vi "Preview the image.vi"() -> ()   [LabVIEW 2018]
uses:
  <userlib>/LabViewDVPCamera/LabViewDVPCamera.lvlib
panel:
  in  "CloseFlg":i32
  out "handle":u32
  out "new picture":picture caption="新图片"
  in  "CameraList":u16(ring) items=["USB2_3M(19)@1112121"]
  in  "Set":bool
  in  "Close":bool
  in  "Open":bool
  in  "ScanCamera":bool
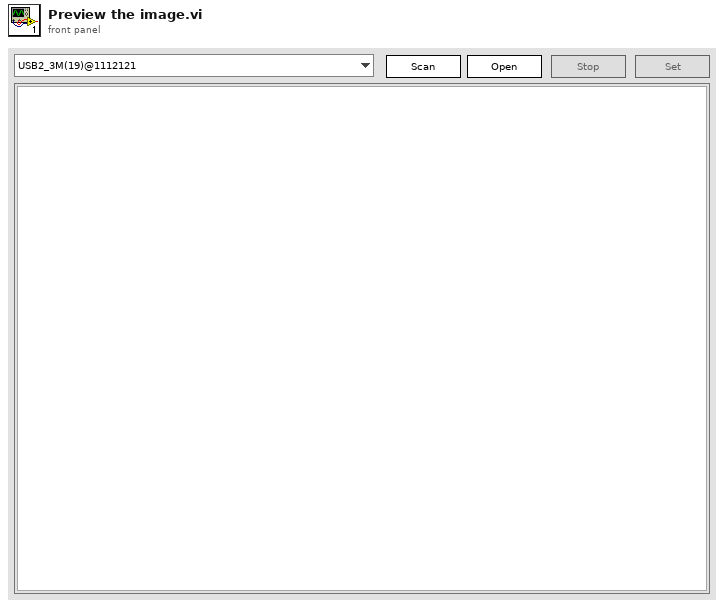
[diagram p1: front panel]
types:
  T1 = enum8{"Enabled", "Disabled", "Disabled and Grayed Out"}
  T2 = typedef "LVStringsAndValuesArrayTypeDef_U16.ctl" = cluster{"String":string, "Value":u16}[]
  T3 = cluster{"image type":i16, "image depth":u8, u8[], "无符号8位数组":u8[], u32[], cluster{u16, u16, u16, u16}}
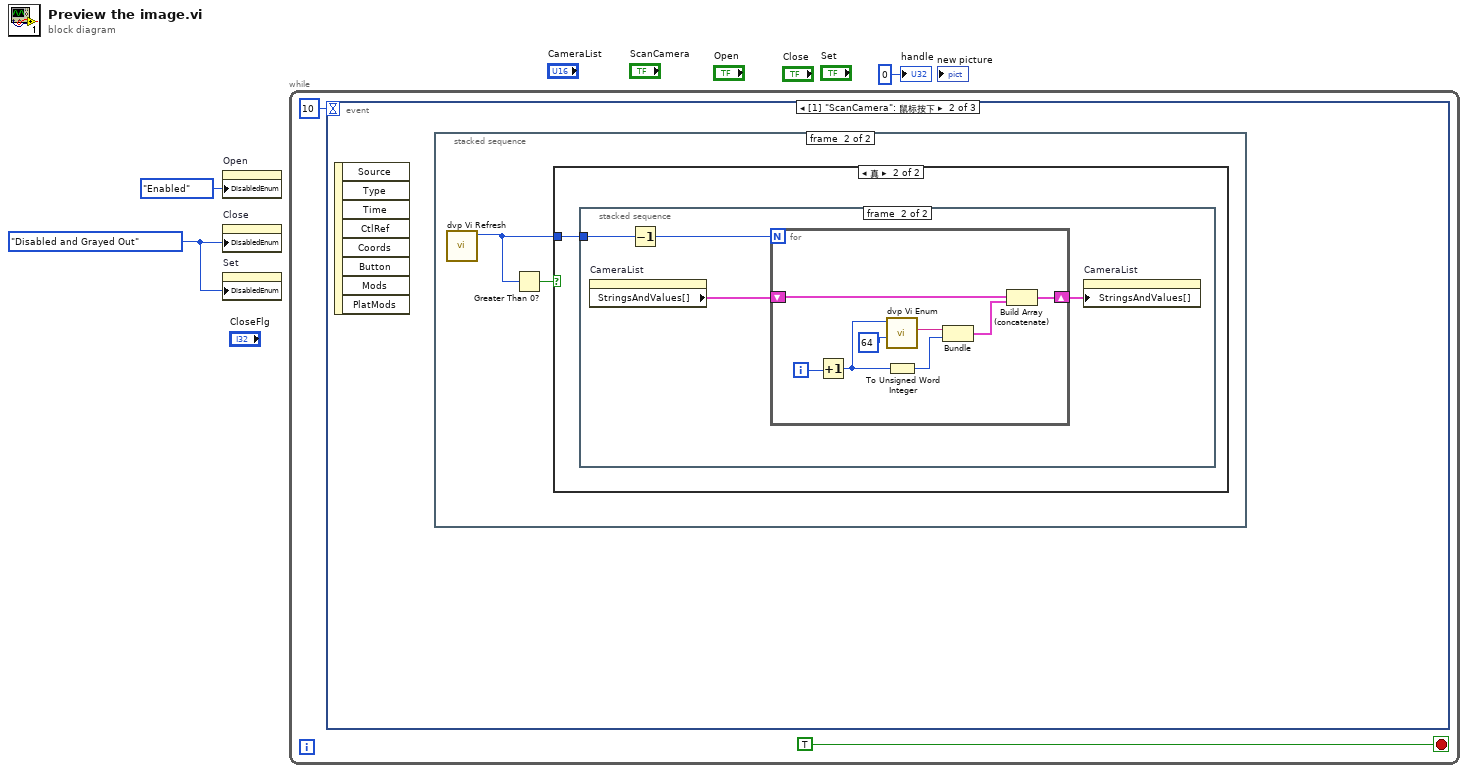
[diagram p0: block diagram]
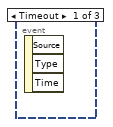
[diagram p2: hidden frame]
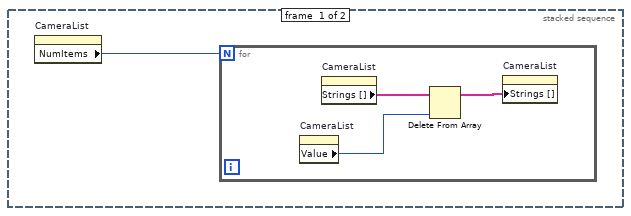
[diagram p3: hidden frame]
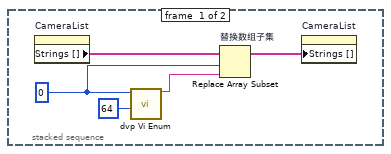
[diagram p5: hidden frame]
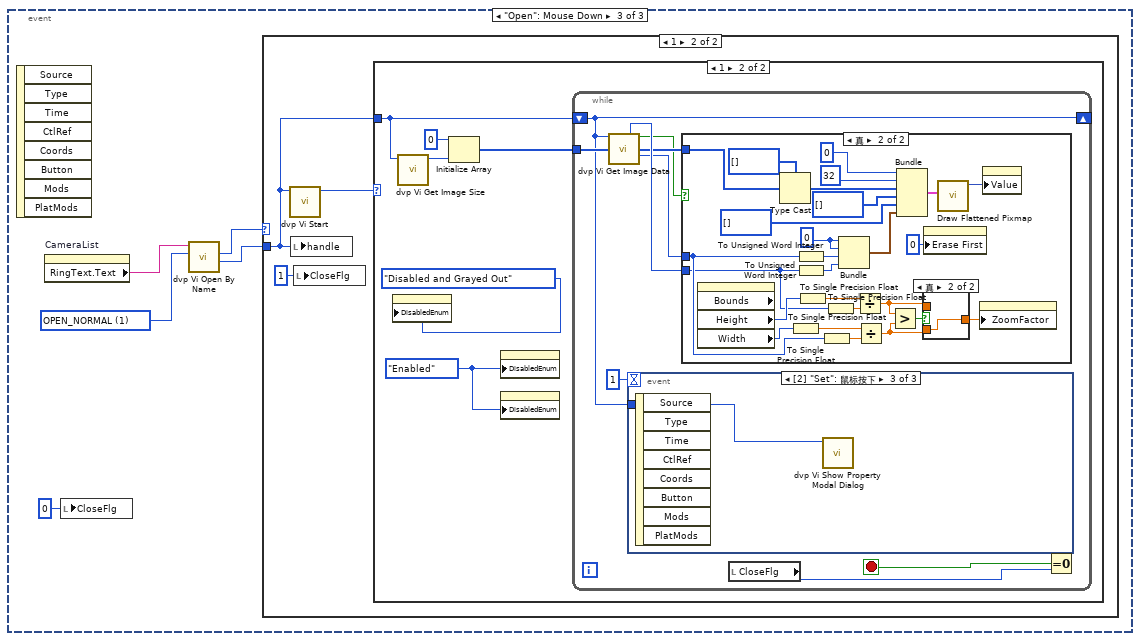
[diagram p6: hidden frame]
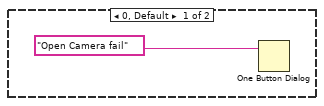
[diagram p7: hidden frame]
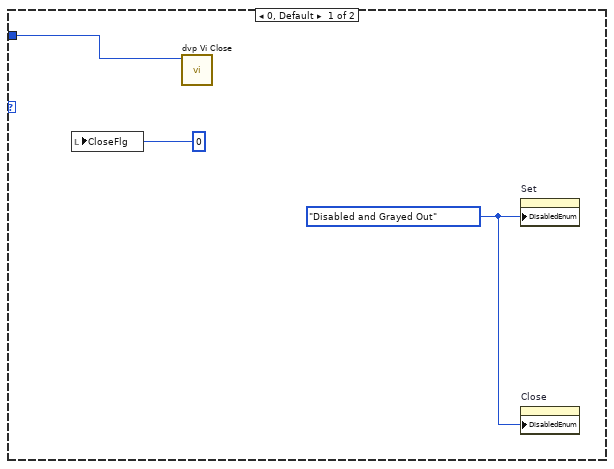
[diagram p8: hidden frame]
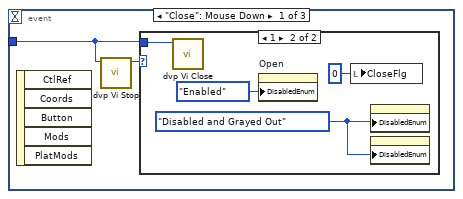
[diagram p9: hidden frame]
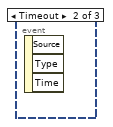
[diagram p11: hidden frame]
diagram:
  w2 = T1."Disabled and Grayed Out" ("禁用")
  n1 = property on="Open" class="Bool"("DisabledEnum"=T1."Enabled" ("禁用")) -> ()  [unwired: 2 in, 2 out]
  n2 = property on="Close" class="Bool"("DisabledEnum"=w2) -> ()  [unwired: 2 in, 2 out]
  n3 = property on="Set" class="Bool"("DisabledEnum"=w2) -> ()  [unwired: 2 in, 2 out]
  n4 = while {
    stop <- TRUE stop-if-true
    n5 = event shown="[1] \"ScanCamera\": 鼠标按下" {
      selector: _ -> [_ _ _]
      dyn-events: _ -> [_ _ _]
      timeout: 10 -> [_ _ _]
      event Timeout {
        n6 = event-data() -> ()  [unwired: 1 in, 3 out]
      }
      event "ScanCamera": Mouse Down {
        n7 = event-data() -> ()  [unwired: 1 in, 8 out]
        n8 = stacked-sequence "清除下拉列表的数据" {
          frame #0 {
            n9 = property on="CameraList" class="Ring (严格)"() -> ("NumItems"=w6:u32)  [unwired: 2 in, 2 out]
            n10 = for {
              N: w6 -> [_]
              n11 = property on="CameraList" class="Ring (严格)"() -> ("Value"=w8:u16)  [unwired: 2 in, 2 out]
              n12 = property on="CameraList" class="Ring (严格)"() -> ("Strings []"=w7:string[])  [unwired: 2 in, 2 out]
              n13 = Delete From Array ("删除数组元素")(array=w7, index=w8) -> (array with subset deleted=w9:string[])  [unwired: 1 in, 1 out]
              n14 = property on="CameraList" class="Ring (严格)"("Strings []"=w9) -> ()  [unwired: 2 in, 2 out]
            }
          }
          frame #1 {
            n15 = call <userlib>:"dvp Vi Refresh.vi"() -> ("pCount out"=w11:u32)  [unwired: 10 in, 1 out]
            n16 = Greater Than 0?(x=w11) -> (x > 0?=w10:bool)
            n17 = case shown="真" w10 {
              tunnel: w11 -> [_ w12]
              frame False {
              }
              frame True {
                n18 = stacked-sequence {
                  tunnel: w12 -> [_ w19]
                  frame #0 {
                    w13 = u32 0 ("index")
                    n19 = property on="CameraList" class="Ring (严格)"() -> ("Strings []"=w16:string[])  [unwired: 2 in, 2 out]
                    n20 = call <userlib>:"dvp Vi Enum.vi"("unSize"=u32 64, "index"=w13) -> ("friendlyName out"=w15:string)  [unwired: 8 in, 1 out]
                    n21 = Replace Array Subset "替换数组子集"(array=w16, new element=w15, index=w13) -> (w17:string[])
                    n22 = property on="CameraList" class="Ring (严格)"("Strings []"=w17) -> ()  [unwired: 2 in, 2 out]
                  }
                  frame #1 {
                    n23 = property on="CameraList" class="Ring (严格)"() -> ("StringsAndValues[]"=w21:T2)  [unwired: 2 in, 2 out]
                    n24 = Decrement(x=w19) -> (x-1=w18:u32)
                    n25 = for {
                      N: w18 -> [_]
                      shift-right: [w28] -> w20
                      shift-left: w21 -> [w26]
                      i -> [w23]
                      n26 = Increment(x=w23) -> (x+1=w22:i32)
                      n27 = call <userlib>:"dvp Vi Enum.vi"("unSize"=u32 64, "index"=w22) -> ("friendlyName out"=w29:string)  [unwired: 8 in, 1 out]
                      n28 = To Unsigned Word Integer(number=w22) -> (unsigned 16bit integer=w25:u16)
                      n29 = Bundle("friendlyName out"=w29, w25) -> (w27:cluster{"friendlyName out":string, u16})  [unwired: 1 in]
                      n30 = Build Array (concatenate)(w26, w27) -> (w28:T2)
                    }
                    n31 = property on="CameraList" class="Ring (严格)"("StringsAndValues[]"=w20) -> ()  [unwired: 2 in, 2 out]
                  }
                }
              }
            }
          }
        }
      }
      event "Open": Mouse Down {
        w32 = u32 1 items=["OPEN_OFFLINE", "OPEN_NORMAL"] ("type")
        n32 = event-data() -> ()  [unwired: 1 in, 8 out]
        n33 = property on="CameraList" class="Ring (严格)"() -> ("RingText.Text"=w31:string)  [unwired: 2 in, 2 out]
        n34 = local write "CloseFlg"(0 ("CloseFlg")) -> ()
        n35 = call <userlib>:"dvp Vi Open By Name.vi"("type"=w32, "friendlyName"=w31) -> ("pHandle out"=w34:u32, "function return"=w33:u32)  [unwired: 7 in, 1 out]
        n36 = case shown="1" w33 {
          tunnel: w34 -> [_ w38]
          frame 0, Default {
            n37 = One Button Dialog(message="Open Camera fail" ("消息")) -> ()  [unwired: 1 in, 1 out]
          }
          frame 1 {
            n38 = call <userlib>:"dvp Vi Start.vi"("handle"=w38) -> ("function return"=w36:u32)  [unwired: 10 in]
            n39 = local write "handle"(w38) -> ()
            n40 = local write "CloseFlg"(1 ("CloseFlg")) -> ()
            n41 = case shown="1" w36 {
              tunnel: w38 -> [w41 w43]
              frame 0, Default {
                w40 = T1."Disabled and Grayed Out" ("禁用")
                n42 = local write "CloseFlg"(0 ("CloseFlg")) -> ()
                n43 = call <userlib>:"dvp Vi Close.vi"("handle"=w41) -> ()  [unwired: 10 in, 1 out]
                n44 = property on="Set" class="Bool"("DisabledEnum"=w40) -> ()  [unwired: 2 in, 2 out]
                n45 = property on="Close" class="Bool"("DisabledEnum"=w40) -> ()  [unwired: 2 in, 2 out]
              }
              frame 1 {
                w47 = T1."Enabled" ("禁用")
                n46 = property on="Open" class="Bool"("DisabledEnum"=T1."Disabled and Grayed Out" ("禁用")) -> ()  [unwired: 2 in, 2 out]
                n47 = call <userlib>:"dvp Vi Get Image Size.vi"("handle"=w43) -> ("function return"=w42:u32)  [unwired: 10 in]
                n48 = Initialize Array(u32 0 ("元素"), w42) -> (w44:u32[])
                n49 = property on="Set" class="Bool"("DisabledEnum"=w47) -> ()  [unwired: 2 in, 2 out]
                n50 = property on="Close" class="Bool"("DisabledEnum"=w47) -> ()  [unwired: 2 in, 2 out]
                n51 = while {
                  shift-right: [w52] -> _
                  shift-left: w43 -> [w52]
                  tunnel: w44 -> [w53]
                  stop <- w55 stop-if-true
                  n52 = call <userlib>:"dvp Vi Get Image Data.vi"("handle"=w52, "pbuffer"=w53) -> ("piHeight out"=w51:i32, "function return"=w48:bool, "pbuffer out"=w49:u32[], "piWidth out"=w50:i32)  [unwired: 9 in, 1 out]
                  n53 = event shown="[2] \"Set\": 鼠标按下" {
                    selector: _ -> [_ _ _]
                    dyn-events: _ -> [_ _ _]
                    timeout: 1 -> [_ _ _]
                    tunnel: w52 -> [w57 _ w63]
                    event "Close": Mouse Down {
                      n54 = event-data() -> ()  [unwired: 1 in, 5 out]
                      n55 = call <userlib>:"dvp Vi Stop.vi"("handle"=w57) -> ("function return"=w58:u32)  [unwired: 10 in]
                      n56 = case shown="1" w58 {
                        tunnel: w57 -> [_ w60]
                        frame 0, Default {
                        }
                        frame 1 {
                          w59 = T1."Disabled and Grayed Out" ("禁用")
                          n57 = call <userlib>:"dvp Vi Close.vi"("handle"=w60) -> ()  [unwired: 10 in, 1 out]
                          n58 = property on="Open" class="Bool"("DisabledEnum"=T1."Enabled" ("禁用")) -> ()  [unwired: 2 in, 2 out]
                          n59 = local write "CloseFlg"(0 ("CloseFlg")) -> ()
                          n60 = property on="Close" class="Bool"("DisabledEnum"=w59) -> ()  [unwired: 2 in, 2 out]
                          n61 = property on="Set" class="Bool"("DisabledEnum"=w59) -> ()  [unwired: 2 in, 2 out]
                        }
                      }
                    }
                    event Timeout {
                      n62 = event-data() -> ()  [unwired: 1 in, 3 out]
                    }
                    event "Set": Mouse Down {
                      n63 = event-data() -> ()  [unwired: 1 in, 8 out]
                      n64 = call <userlib>:"dvp Vi Show Property Modal Dialog.vi"("handle"=w63) -> ()  [unwired: 10 in, 1 out]
                    }
                  }
                  n65 = case shown="真" w48 {
                    tunnel: w49 -> [_ w67]
                    tunnel: w50 -> [_ w71]
                    tunnel: w51 -> [_ w70]
                    frame False {
                    }
                    frame True {
                      w87 = u16 0
                      n66 = property on="new picture" class="Pict" props=["Bounds", "Height", "Width"]() -> ("Height"=w80:u32, "Width"=w79:u32)  [unwired: 2 in, 3 out]
                      n67 = Type Cast(type=u8[] [], x=w67) -> (*(type *) &x=w66:u8[])
                      n68 = To Single Precision Float(number=w79) -> (single precision float=w72:sgl)
                      n69 = To Unsigned Word Integer(number=w71) -> (unsigned 16bit integer=w86:u16)
                      n70 = To Unsigned Word Integer(number=w70) -> (unsigned 16bit integer=w85:u16)
                      n71 = To Single Precision Float(number=w80) -> (single precision float=w78:sgl)
                      n72 = To Single Precision Float(number=w71) -> (single precision float=w76:sgl)
                      n73 = To Single Precision Float(number=w70) -> (single precision float=w77:sgl)
                      n74 = Bundle ("图像尺寸")(w87, w87, w86, w85) -> (w84:cluster{u16, u16, u16, u16})  [unwired: 1 in]
                      n75 = Divide(x=w78, y=w77) -> (x/y=w74:sgl)
                      n76 = Divide(x=w72, y=w76) -> (x/y=w73:sgl)
                      n77 = Greater?(x=w74, y=w73) -> (0:w75:bool)
                      n78 = Bundle ("图像数据")("image type"=i16 0, "image depth"=u8 32, w66, "无符号8位数组"=u8[] [], u32[] [], w84) -> (w68:T3)  [unwired: 1 in]
                      n79 = case shown="真" w75 {
                        tunnel: w74 -> [w90 _]
                        tunnel: w73 -> [_ w91]
                        tunnel: [w90 w91] -> w69
                        frame False {
                        }
                        frame True {
                        }
                      }
                      n80 = property on="new picture" class="Pict"("Erase First"=u8 0 ("画前清除图片")) -> ()  [unwired: 2 in, 2 out]
                      n81 = call <vilib>:"Draw Flattened Pixmap.vi"("image data"=w68) -> ("new picture"=w81:picture)  [unwired: 8 in]
                      n82 = property on="new picture" class="Pict"("ZoomFactor"=w69) -> ()  [unwired: 2 in, 2 out]
                      n83 = property on="new picture" class="Pict"("Value"=w81) -> ()  [unwired: 2 in, 2 out]
                    }
                  }
                  n84 = local read "CloseFlg"() -> (w54:i32)
                  n85 = Equal To 0?(x=w54) -> (x = 0?=w55:bool)
                }
              }
            }
          }
        }
      }
    }
  }
  "handle" <- u32 0 ("handle")
